vi "SimpleStreamFullSpectrumFromStorageExample.vi"() -> ()   [LabVIEW 2016]
uses:
  h.Library/ACQ/CTL/h.ACQ.SpectralData.ctl
  h.Library/ACQ/CTL/h.ACQ.Spectrum.ctl
  h.Library/COMM/CTL/h.COMM.Socket Type.ctl
  h.Library.lvlib
panel:
  out "Number of Spectra Returned":i32
  out "Serial Numbers":u64[](array[numeric])
  out "Spectral Data":T1 {"Spectrum"."Spectrum, db" format="%_8g"}
  in  "IP Address":string="10.0.41.3"
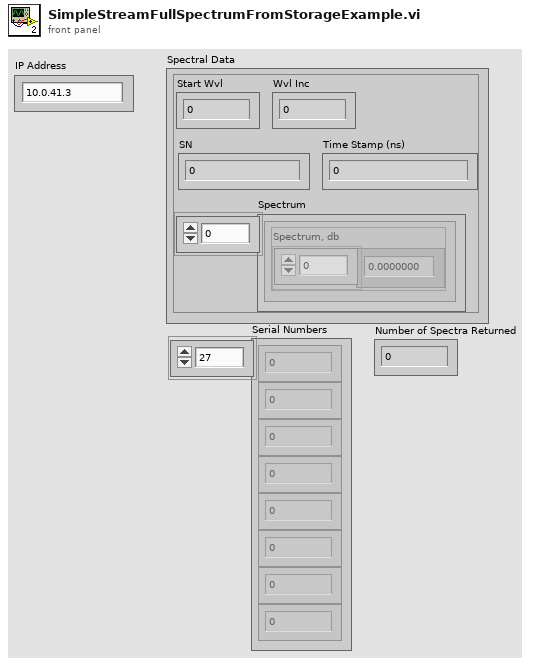
[diagram p1: front panel]
types:
  T1 = typedef "h.Library.lvlib/h.ACQ.SpectralData.ctl" = cluster{"Spectrum":T2[], "Start Wvl":dbl, "Wvl Inc":dbl, "SN":u64, "Time Stamp (ns)":u64}
  T2 = typedef "h.Library.lvlib/h.ACQ.Spectrum.ctl" = cluster{"Spectrum, db":dbl[]}
  T3 = typedef "h.Library.lvlib/h.COMM.Socket Type.ctl" = u16
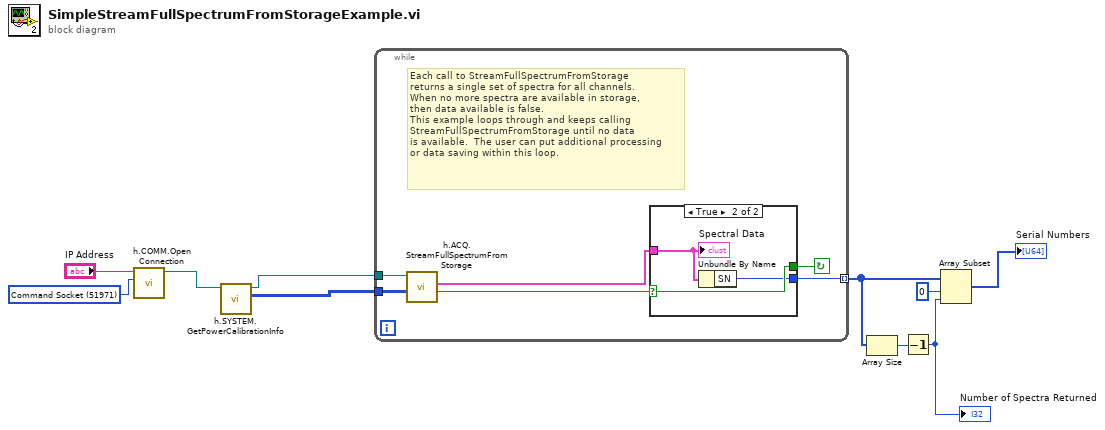
[diagram p0: block diagram]
diagram:
  w9 = T3 51971 items=["Command Socket"=51971, "Streaming Peak Data Socket"=51972, "Streaming Spectral Data Socket"=51973] ("Port")
  n1 = call "h.COMM.Open Connection.vi"("Port"=w9, "Address"="IP Address") -> ("Connection ID"=w3:refnum<k5>)  [unwired: 8 in, 1 out]
  n2 = call "h.SYSTEM.GetPowerCalibrationInfo.vi"("Connection ID"=w3) -> ("power scales and offsets"=w1:i32[][], "Connection ID out"=w2:refnum<k5>)  [unwired: 8 in, 1 out]
  n3 = while {
    tunnel: w2 -> [w16]
    tunnel: [w12] -> w6 mode=indexing
    tunnel: w1 -> [w11]
    stop <- w13 continue-if-true
    # "Each call to StreamFullSpectrumFromStorage\nreturns a single set of spectra for all channels.\nWhen no more spectra are available in storage,\nthen data available is false.\nThis example loops through and keeps calling\nStreamFullSpectrumFromStorage until no data\nis available.  The user can put additional processing \nor data saving within this loop."
    n4 = call "h.ACQ.StreamFullSpectrumFromStorage.vi"("power scales and offsets"=w11, "Connection ID In"=w16) -> ("Data Available"=w15:bool, "Spectral Data"=w14:T1)  [unwired: 6 in, 2 out]
    n5 = case shown="True" w15 {
      selector: w15 -> [w17 w20]
      tunnel: w14 -> [_ w19]
      tunnel: [w17 w20] -> w13
      tunnel: [_ w18] -> w12
      frame False {
      }
      frame True {
        n6 = Unbundle By Name(w19) -> ("SN"=w18:u64)
        "Spectral Data" <- w19
      }
    }
  }
  n7 = Array Size(array=w6) -> (size(s)=w8:i32)
  n8 = Decrement(x=w8) -> (x-1=w5:i32)
  "Number of Spectra Returned" <- w5
  n9 = Array Subset(array=w6, index=0, length=w5) -> (→"Serial Numbers":u64[])
